vi "SALimitConfigureData.vi"(7 "DataArray":dbl[](array[numeric])=[0.0] format="%.2p", 8 "error in (no error)":errorcluster {"code" format="%.0x"}, 10 "RepCapIdentifier":string="Limit1" caption="RepCapIdentifier (Limit1)", 11 "instrument handle":refnum<k15>) -> (0 "error out":errorcluster {"code" format="%.0x"}, 3 "instrument handle out":refnum<k15>)   [LabVIEW 2009, in "Keysight XSAn.lvlib"]
doc: "Defines the limit line values, and destroys all existing data. \n\nSupported Models: M9290A, N8973B, N8974B, N8975B, N8976B, N9000A, N9000B, N9010A, N9010B, N9020A, N9020B, N9030A, N9030B, N9038A, N9040B, N9041B, SPN9003A, SPN9026A"
uses:
  <instrlib>/Keysight XSAn/Keysight XSAn.lvlib
  AgXSAn.dll
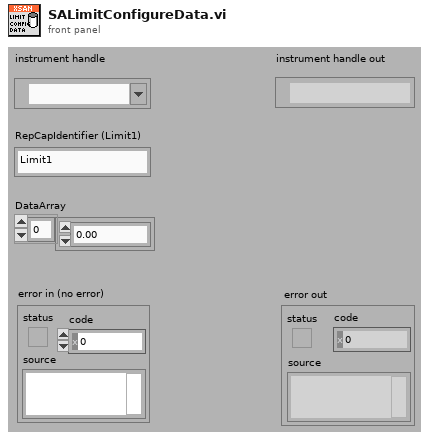
[diagram p1: front panel]
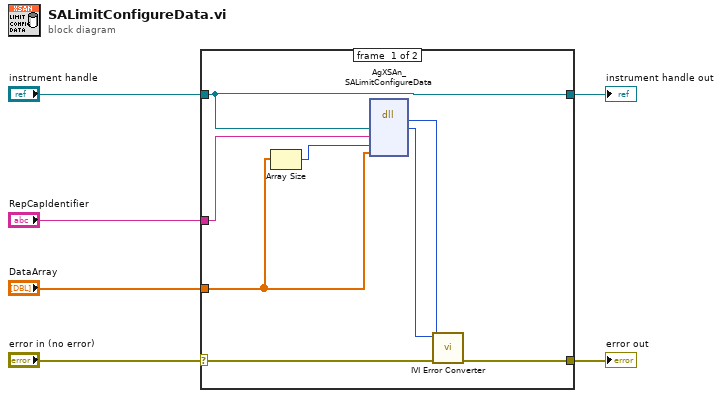
[diagram p0: block diagram]
diagram:
  n1 = case shown="No Error" "error in (no error)" {
    selector: "error in (no error)" -> [w12 w16]
    tunnel: [w11 w16] -> w6
    tunnel: "instrument handle" -> [w9 w15]
    tunnel: "RepCapIdentifier" -> [w10 _]
    tunnel: "DataArray" -> [w8 _]
    tunnel: [w9 w15] -> w1
    frame #0 {
      n2 = Array Size(array=w8) -> (size(s)=w7:i32)
      n3 = dll-call lib="AgXSAn**.dll" fn="AgXSAn_SALimitConfigureData"("Vi"=w9, "RepCapIdentifier"=w10, "DataArrayBufferSize"=w7, "DataArray"=w8) -> (w13:i32, "Vi"=w14:u32)  [unwired: 6 in, 2 out]
      n4 = call <instrlib>:"IVI Error Converter.vi"("error in (no error)"=w12, "IVI error code (0)"=w13, "instrument handle"=w14) -> ("error out"=w11:errorcluster)  [unwired: 7 in, 1 out]
    }
    frame #1 {
    }
  }
  "error out" <- w6
  "instrument handle out" <- w1
